vi "Size.vi"(0 "State In":T1={"Input Type"=variant(dbl 0.0), "Width"=0, "Typedef Name"="", "Value Type"=variant, "Selection"=0, "Options"=[], "Selections"=[], "Display Selections"=[], "Element Names"=[], "Typedef Name Width"=0, "Display Selection Width"=[], "Code Generated"=FALSE}, 1 "XRef":refnum<vi>, 3 "Bounds":T8) -> (2 "State Out":T1={"Input Type"=variant(dbl 0.0), "Width"=0, "Typedef Name"="", "Value Type"=variant, "Selection"=0, "Options"=[], "Selections"=[], "Display Selections"=[], "Element Names"=[], "Typedef Name Width"=0, "Display Selection Width"=[], "Code Generated"=FALSE}, 4 "Reply":string[](array[string]))   [LabVIEW 2015, in "Read-Write-Signals.xnode"]
doc: "This ability VI is called by LabVIEW after the user resizes the XNode. Bounds is a recatangle whose coordinates are given relative to the old top-left corner of the XNode. You must either return a UpdateImageAndBounds reply or not return anything, otherwise LabVIEW will generate an error. If you return UpdateImageAndBounds, you may also return other reply strings.\n\nDefault behavior: None.\n\nThis ability does not provide UI and OS messages are not handled.\n\nSee also: GetGrowInfo"
uses:
  Read-Write-Signals.xnode
  State.ctl
  Read-Write-Signals Item.ctl
  Read-Write-Signals Sub Item.ctl
  Read-Write-Signals Sub Item Type.ctl
  Read-Write-Signals Selection.ctl
  Read-Write-Signals Display Selection.ctl
  <vilib>/XNodeSupport/XNodeInt.ctl
  <vilib>/XNodeSupport/NI_XNodeSupport.lvlib
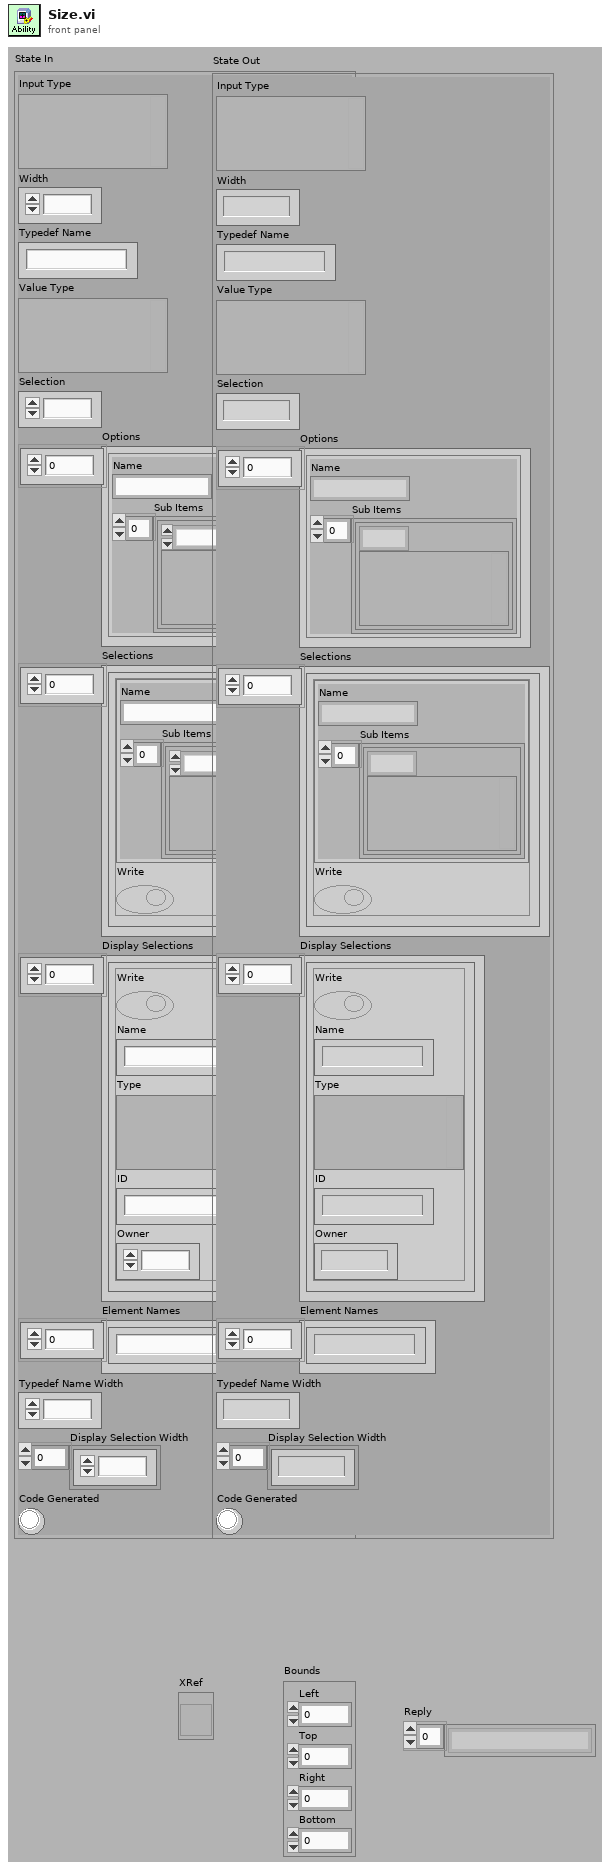
[diagram p1: front panel]
types:
  T1 = typedef "Read-Write-Signals.xnode/State.ctl" = cluster{"Input Type":variant, "Width":i32, "Typedef Name":string, "Value Type":variant, "Selection":i32, "Options":T2[], "Selections":T5[], "Display Selections":T6[], "Element Names":string[], "Typedef Name Width":i32, "Display Selection Width":i32[], "Code Generated":bool}
  T2 = typedef "Read-Write-Signals Item.ctl" = cluster{"Name":string, "Sub Items":T3[]}
  T3 = typedef "Read-Write-Signals Sub Item.ctl" = cluster{"Type":T4, "Value":variant}
  T4 = typedef "Read-Write-Signals Sub Item Type.ctl" = enum8{"Cluster Element", "Array Element", "Subarray"}
  T5 = typedef "Read-Write-Signals Selection.ctl" = cluster{"Item":T2, "Write":bool}
  T6 = typedef "Read-Write-Signals Display Selection.ctl" = cluster{"Write":bool, "Name":string, "Type":variant, "ID":string, "Owner":i32}
  T7 = typedef "NI_XNodeSupport.lvlib/XNodeInt.ctl" = i32
  T8 = cluster{"Left":T7, "Top":T7, "Right":T7, "Bottom":T7}
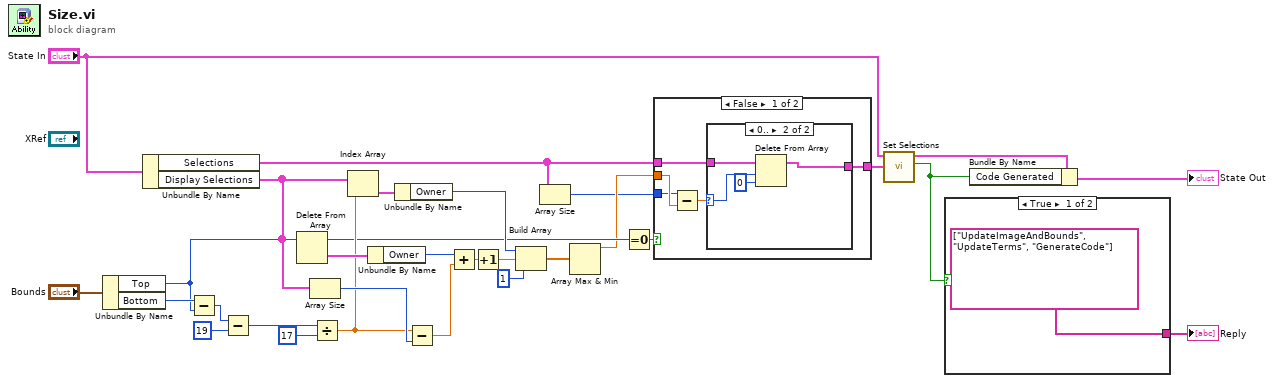
[diagram p0: block diagram]
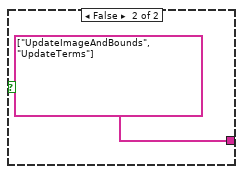
[diagram p2: hidden frame]
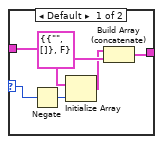
[diagram p3: hidden frame]
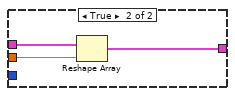
[diagram p4: hidden frame]
diagram:
  n1 = Unbundle By Name("Bounds") -> ("Top"=w13:T7, "Bottom"=w29:T7)
  n2 = Unbundle By Name("State In") -> ("Selections"=w9:T5[], "Display Selections"=w8:T6[])
  n3 = Subtract(x=w29, y=w13) -> (x-y=w28:T7)
  n4 = Subtract(x=w28, y=T7 19) -> (x-y=w27:T7)
  n5 = Delete From Array(array=w8) -> (deleted portion=w23:T6)  [unwired: 2 in, 1 out]
  n6 = Array Size(array=w8) -> (size(s)=w22:i32)
  n7 = Divide(x=w27, y=T7 17) -> (x/y=w21:dbl)
  n8 = Index Array(array=w8, index=w21) -> (element=w24:T6)
  n9 = Unbundle By Name(w23) -> ("Owner"=w20:i32)
  n10 = Unbundle By Name(w24) -> ("Owner"=w16:i32)
  n11 = Subtract(x=w21, y=w22) -> (x-y=w19:dbl)
  n12 = Add(x=w20, y=w19) -> (x+y=w18:dbl)
  n13 = Increment(x=w18) -> (x+1=w17:dbl)
  n14 = Build Array(w16, w17, 1) -> (w14:dbl[])
  n15 = Array Size(array=w9) -> (size(s)=w10:i32)
  n16 = Array Max & Min(array=w14) -> (max value=w11:dbl)  [unwired: 3 out]
  n17 = Equal To 0?(x=w13) -> (x = 0?=w12:bool)
  n18 = case shown="False" w12 {
    tunnel: [w31 w46] -> w5
    tunnel: w9 -> [w32 w47]
    tunnel: w11 -> [w34 w45]
    tunnel: w10 -> [w33 _]
    frame False {
      n19 = Subtract(x=w33, y=w34) -> (x-y=w30:dbl)
      n20 = case shown="0.." w30 {
        selector: w30 -> [w39 w41]
        tunnel: w32 -> [w40 w44]
        tunnel: [w37 w43] -> w31
        frame Default {
          n21 = Negate(x=w39) -> (-x=w36:i32)
          n22 = Initialize Array(T5 {"Item"={"Name"="", "Sub Items"=[]}, "Write"=FALSE} ("Selection"), w36) -> (w38:T5[])
          n23 = Build Array (concatenate)(w38, w40) -> (w37:T5[])
        }
        frame 0.. {
          n24 = Delete From Array(array=w44, length=w41, index=0) -> (array with subset deleted=w43:T5[])  [unwired: 1 out]
        }
      }
    }
    frame True {
      n25 = Reshape Array(w47, w45) -> (w46:T5[])
    }
  }
  n26 = call "Set Selections.vi"("Selections"=w5, "State in"="State In") -> ("All Valid"=w1:bool, "State out"=w3:T1)  [unwired: 8 in]
  n27 = case shown="True" w1 {
    tunnel: [string[] ["UpdateImageAndBounds", "UpdateTerms", "GenerateCode"] ("Reply") string[] ["UpdateImageAndBounds", "UpdateTerms"] ("Reply")] -> w6
    frame True {
    }
    frame False {
    }
  }
  "Reply" <- w6
  n28 = Bundle By Name(cluster=w3, "Code Generated"=w1) -> (→"State Out":T1)
